vi "Heila IQ Login.vi"(8 "error in (no error)":errorcluster, 11 "Modbus master in":refnum<class "Modbus Master.lvclass">) -> (0 "error out":errorcluster, 3 "Modbus master out":refnum<class "Modbus Master.lvclass">)   [LabVIEW 2017]
uses:
  <vilib>/Modbus/master/Modbus Master.lvclass
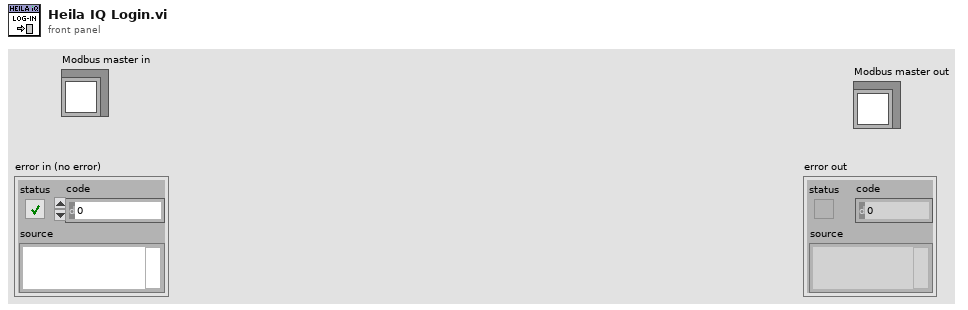
[diagram p1: front panel]
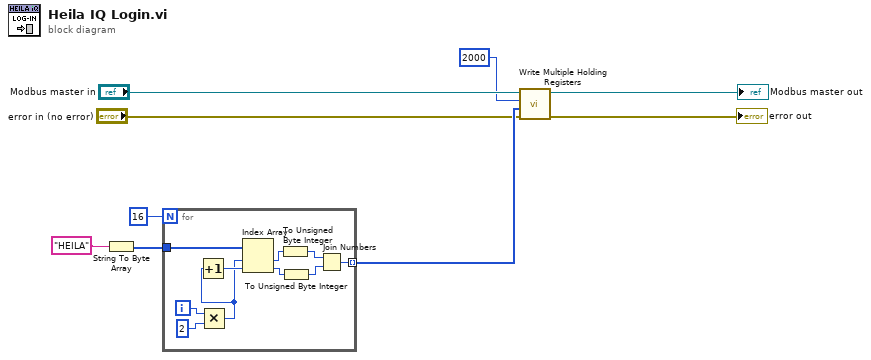
[diagram p0: block diagram]
diagram:
  n1 = String To Byte Array(string="HEILA") -> (unsigned byte array=w9:u8[])
  n2 = for {
    N: 16 -> [_]
    tunnel: w9 -> [w19]
    tunnel: [w18] -> w7 mode=indexing
    i -> [w14]
    n3 = Multiply(x=w14, y=2) -> (x*y=w15:i32)
    n4 = Increment(x=w15) -> (x+1=w16:i32)
    n5 = Index Array(array=w19, index #1=w15, index #2=w16) -> (element #1=w13:u8, element #2=w11:u8)
    n6 = To Unsigned Byte Integer(number=w13) -> (unsigned 8bit integer=w12:u8)
    n7 = To Unsigned Byte Integer(number=w11) -> (unsigned 8bit integer=w10:u8)
    n8 = Join Numbers(hi=w12, lo=w10) -> ((hi.lo)=w18:u16)
  }
  n9 = call-dynamic "Write Multiple Holding Registers.vi"("error in (no error)"="error in (no error)", "holding register values"=w7, "starting address"=u16 2000, "Modbus master in"="Modbus master in") -> ("error out"=→"error out":errorcluster, "Modbus master out"=→"Modbus master out":refnum<class "Modbus Master.lvclass">)  [unwired: 6 in]
